vi "unicastTiming.vi"(8 "error in (no error)":errorcluster, 10 "Latency in":u32, 11 "DynamicFrameBuilder in":refnum<class "DynamicFrameBuilder.lvclass">) -> (0 "error out":errorcluster, 1 "WaitForRxTimeout":u16, 2 "Latency out":u32, 3 "DynamicFrameBuilder out":refnum<class "DynamicFrameBuilder.lvclass">)   [LabVIEW 2016, in "RTModbus.lvlib" / "DynamicFrameBuilder.lvclass"]
uses:
  DynamicFrameBuilder.lvclass
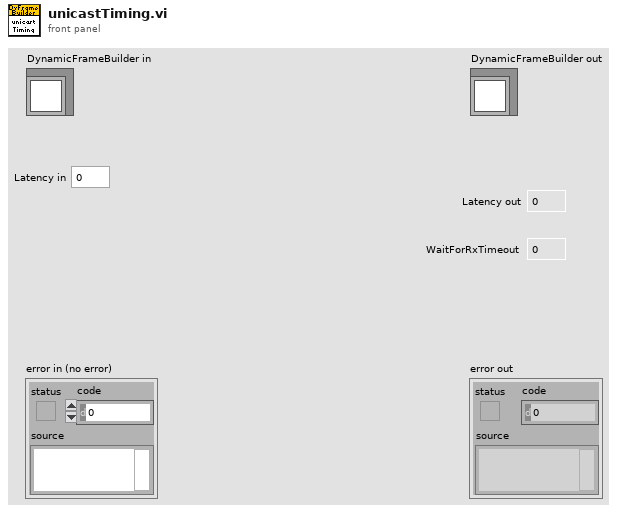
[diagram p1: front panel]
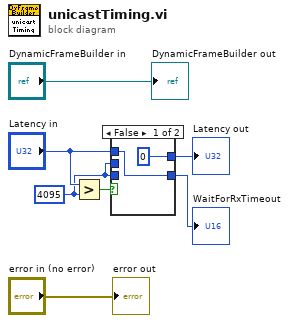
[diagram p0: block diagram]
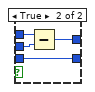
[diagram p2: hidden frame]
diagram:
  w2 = u32 4095 ("y")
  n1 = Greater?(x="Latency in", y=w2) -> (0:w5:bool)
  n2 = case shown="False" w5 {
    tunnel: "Latency in" -> [w9 w12]
    tunnel: [w9 w13] -> w3
    tunnel: w2 -> [_ w13]
    tunnel: w2 -> [_ w11]
    tunnel: [u32 0 w10] -> w1
    frame False {
    }
    frame True {
      n3 = Subtract(x=w12, y=w11) -> (x-y=w10:u32)
    }
  }
  "WaitForRxTimeout" <- w3
  "Latency out" <- w1
  "error out" <- "error in (no error)"
  "DynamicFrameBuilder out" <- "DynamicFrameBuilder in"
